vi "Handle Error.vi"(8 "error in (no error)":errorcluster, 11 "TestLNA in":refnum<class "TestLNA.lvclass">) -> (0 "error out":errorcluster, 2 "stop actor?":bool=TRUE, 3 "TestLNA out":refnum<class "TestLNA.lvclass">)   [LabVIEW 2014, in "TestLNA.lvlib" / "TestLNA.lvclass"]
doc: "(<B>Filename</B>: Actor Framework.lvlib:Actor.lvclass:Handle Error.vi)\n\nDefines how the actor handles an error that occurred while processing a message.\n\nBy default, this method does nothing except stop the actor. This method also treats error code 43 (coming from <B>error in</B>) as a sign that the actor shut down normally. In this situation, the Handle Error method does not return the error on <B>error out</B>, meaning the actor's caller will not receive it. All other error codes will be returned on <B>error out</B>.\n\nA descendant class may override this method to change this behavior."
uses:
  TestLNA.lvclass
  TestLNA.lvclass/TestLNA.ctl
  LNA Messages/LNA Return Message Msg/LNA Return Message Msg.lvclass
  <vilib>/ActorFramework/Actor/Actor.lvclass/Actor.ctl
  <vilib>/ActorFramework/Message Enqueuer/Message Enqueuer.lvclass/Message Enqueuer.ctl
  <vilib>/ActorFramework/Message Enqueuer/Init from Existing Queue.vi
  <vilib>/ActorFramework/Message Enqueuer/Message Enqueuer.lvclass
  CSPP_Core/Actors/CS++BaseActor/CS++BaseActor.lvclass
  <vilib>/ActorFramework/Actor/Actor.lvclass
  CSPP_LNA/CS++LNA.lvlib
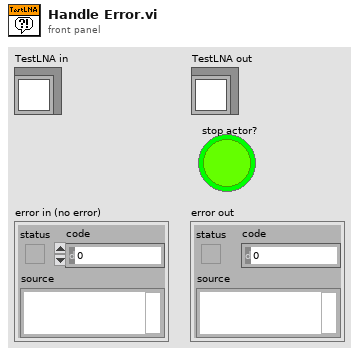
[diagram p1: front panel]
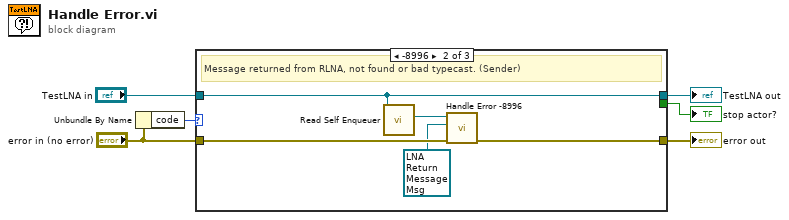
[diagram p0: block diagram]
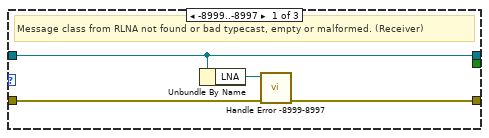
[diagram p2: hidden frame]
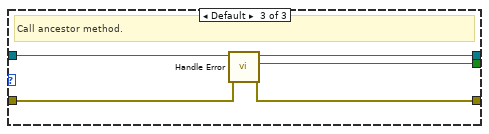
[diagram p3: hidden frame]
diagram:
  n1 = Unbundle By Name("error in (no error)") -> ("code"=w4:i32)
  n2 = case shown="-8996" w4 {
    tunnel: [w8 w11 w18] -> w1
    tunnel: [w10 w15 w17] -> w2
    tunnel: "error in (no error)" -> [w7 w13 w19]
    tunnel: "TestLNA in" -> [w10 w15 w20]
    tunnel: [_ _ w16] -> w3
    frame -8999..-8997 {
      # "Message class from RLNA not found or bad typecast, empty or malformed. (Receiver)"
      n3 = Unbundle By Name(w10) -> ("LNA"=w9:refnum<class "Message Enqueuer.lvclass">)
      n4 = call "Handle Error -8999-8997.vi"("Tx Error"=w7, "Message Enqueuer in"=w9) -> ("Error Out"=w8:errorcluster)  [unwired: 9 in]
    }
    frame -8996 {
      # "Message returned from RLNA, not found or bad typecast. (Sender)"
      n5 = call <vilib>:"Read Self Enqueuer.vi"("Actor"=w15) -> ("Self Enqueuer"=w14:refnum<class "Message Enqueuer.lvclass">)  [unwired: 10 in]
      n6 = call "Handle Error -8996.vi"("Tx Error"=w13, "LNA Return Message Msg"=refnum<class "LNA Return Message Msg.lvclass"> refnum ("TestLNA.lvlib:LNA Return Message Msg.lvclass"), "Message Enqueuer in"=w14) -> ("Error Out"=w11:errorcluster)  [unwired: 8 in]
    }
    frame Default {
      # "Call ancestor method."
      n7 = call-parent "Handle Error.vi"("error in (no error)"=w19, "CS++BaseActor in"=w20) -> ("error out"=w18:errorcluster, "stop actor?"=w16:bool, "CS++BaseActor out"=w17:refnum<class "TestLNA.lvclass">)  [unwired: 7 in]
    }
  }
  "TestLNA out" <- w2
  "error out" <- w1
  "stop actor?" <- w3
